vi "svx_Polar_Get_Annotation.vi"(7 "Polar Plot":refnum<vi>, 11 "data":T1) -> (2 "Array":cluster{dbl, dbl}[](array[cluster]), 3 "marker value":dbl[](array[numeric]))   [LabVIEW 2017, in "SVX Polar Plot.xctl"]
uses:
  <vilib>/addons/_XControls/Polar Plot/SVX Polar Plot.xctl
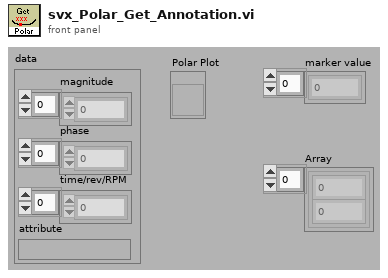
[diagram p1: front panel]
types:
  T1 = cluster{"magnitude":dbl[], "phase":dbl[], "time/rev/RPM":dbl[], "attribute":variant}
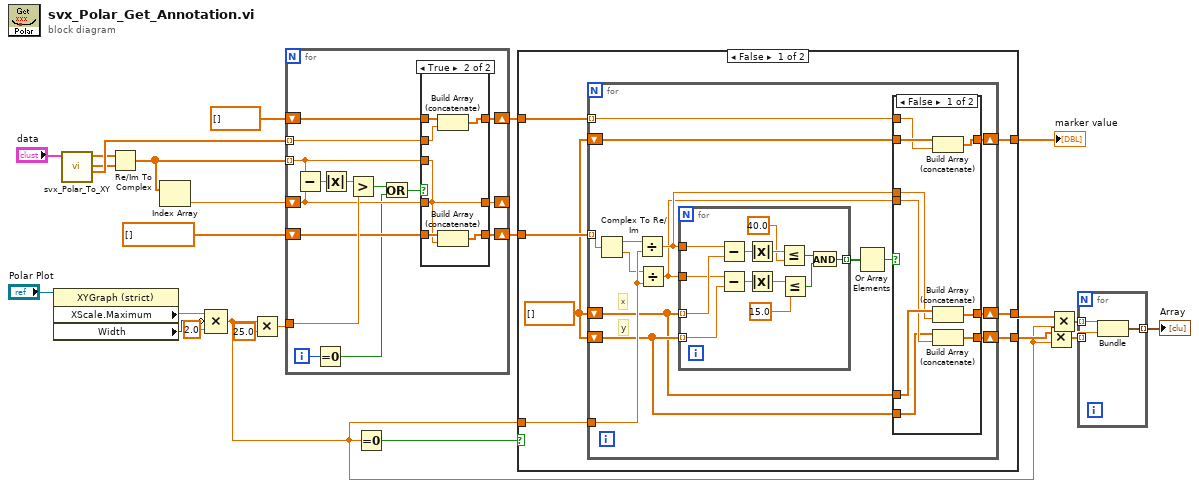
[diagram p0: block diagram]
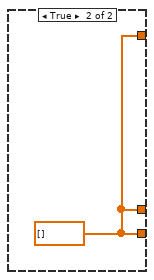
[diagram p3: hidden frame]
diagram:
  n1 = property class="XYGraph (strict)"(reference="Polar Plot") -> ("XScale.Maximum"=w24:dbl, "Width"=w23:u32)  [unwired: 1 in, 2 out]
  n2 = call <vilib>:"svx_Polar_To_XY.vi"("polar plot"="data") -> ("time/rev/RPM"=w5:dbl[], "y"=w3:dbl[], "x"=w4:dbl[])  [unwired: 7 in, 1 out]
  n3 = Re/Im To Complex(1:w3, 2:w4) -> (0:w20:cdb[])
  n4 = Index Array(array=w20) -> (element=w21:cdb)  [unwired: 1 in]
  n5 = Compound Arithmetic op=MULTIPLY(w24, invert w23, 2.0 ("value")) -> (w13:dbl)
  n6 = Multiply(x=w13, y=25.0) -> (x*y=w18:dbl)
  n7 = for {
    tunnel: w20 -> [w36] mode=indexing
    shift-right: [w35] -> _
    shift-left: w21 -> [w34]
    tunnel: w18 -> [w37]
    shift-right: [w32] -> w9
    shift-left: cdb[] [] ("r * e^(i*theta)") -> [w33]
    tunnel: w5 -> [w29] mode=indexing
    shift-right: [w30] -> w10
    shift-left: dbl[] [] -> [w31]
    i -> [w28]
    n8 = Subtract(x=w36, y=w34) -> (x-y=w39:cdb)
    n9 = Equal To 0?(x=w28) -> (x = 0?=w25:bool)
    n10 = Absolute Value(x=w39) -> (abs(x)=w38:dbl)
    n11 = Greater?(x=w38, y=w37) -> (0:w27:bool)
    n12 = Or(x=w27, y=w25) -> (x .or. y?=w26:bool)
    n13 = case shown="True" w26 {
      tunnel: w36 -> [_ w47]
      tunnel: [w42 w47] -> w35
      tunnel: w34 -> [w42 _]
      tunnel: w33 -> [w41 w48]
      tunnel: [w41 w46] -> w32
      tunnel: w31 -> [w40 w45]
      tunnel: [w40 w43] -> w30
      tunnel: w29 -> [_ w44]
      frame False {
      }
      frame True {
        n14 = Build Array (concatenate)(w45, w44) -> (w43:dbl[])
        n15 = Build Array (concatenate)(w48, w47) -> (w46:cdb[])
      }
    }
  }
  n16 = Equal To 0?(x=w13) -> (x = 0?=w16:bool)
  n17 = case shown="False" w16 {
    tunnel: w9 -> [w55 _]
    tunnel: w13 -> [w54 _]
    tunnel: [w53 w96] -> w15
    tunnel: [w52 w96] -> w14
    tunnel: w10 -> [w51 _]
    tunnel: [w49 w96] -> w6
    frame False {
      w50 = dbl[] []
      n18 = for {
        tunnel: w55 -> [w59] mode=indexing
        tunnel: w54 -> [w70]
        shift-right: [w65] -> w53
        shift-left: w50 -> [w66]
        shift-right: [w64] -> w52
        shift-left: w50 -> [w67]
        tunnel: w51 -> [w56] mode=indexing
        shift-right: [w58] -> w49
        shift-left: w50 -> [w57]
        # "y"
        # "x"
        n19 = Complex To Re/Im(x + iy=w59) -> (x=w63:dbl, y=w61:dbl)
        n20 = Divide(x=w63, y=w70) -> (x/y=w62:dbl)
        n21 = Divide(x=w61, y=w70) -> (x/y=w60:dbl)
        n22 = for {
          tunnel: w62 -> [w95]
          tunnel: w60 -> [w93]
          tunnel: w66 -> [w94] mode=indexing
          tunnel: w67 -> [w92] mode=indexing
          tunnel: [w83] -> w69 mode=indexing
          n23 = Subtract(x=w95, y=w94) -> (x-y=w91:dbl)
          n24 = Subtract(x=w93, y=w92) -> (x-y=w90:dbl)
          n25 = Absolute Value(x=w91) -> (abs(x)=w89:dbl)
          n26 = Absolute Value(x=w90) -> (abs(x)=w88:dbl)
          n27 = Less Or Equal?(x=w89, y=40.0) -> (x <= y?=w85:bool)
          n28 = Less Or Equal?(x=w88, y=15.0) -> (x <= y?=w84:bool)
          n29 = And(x=w85, y=w84) -> (x .and. y?=w83:bool)
        }
        n30 = Or Array Elements(Boolean array=w69) -> (logical OR=w68:bool)
        n31 = case shown="False" w68 {
          tunnel: w62 -> [w77 _]
          tunnel: w60 -> [w75 _]
          tunnel: w67 -> [w74 w81]
          tunnel: w66 -> [w79 w82]
          tunnel: [w78 w82] -> w65
          tunnel: [w76 w81] -> w64
          tunnel: [w73 w80] -> w58
          tunnel: w57 -> [w72 w80]
          tunnel: w56 -> [w71 _]
          frame False {
            n32 = Build Array (concatenate)(w72, w71) -> (w73:dbl[])
            n33 = Build Array (concatenate)(w79, w77) -> (w78:dbl[])
            n34 = Build Array (concatenate)(w74, w75) -> (w76:dbl[])
          }
          frame True {
            # "overlap"
          }
        }
      }
    }
    frame True {
      w96 = dbl[] []
    }
  }
  "marker value" <- w6
  n35 = Multiply(x=w14, y=w13) -> (x*y=w8:dbl[])
  n36 = Multiply(x=w15, y=w13) -> (x*y=w7:dbl[])
  n37 = for {
    tunnel: w7 -> [w99] mode=indexing
    tunnel: w8 -> [w98] mode=indexing
    tunnel: [w97] -> w12 mode=indexing
    n38 = Bundle(w99, w98) -> (w97:cluster{dbl, dbl})  [unwired: 1 in]
  }
  "Array" <- w12
